vi "RefreshSystemConfigurationUI.vi"(8 "error in (no error)":errorcluster, 11 "SystemSetup in":refnum<class "SystemSetup.lvclass">) -> (0 "error out":errorcluster, 3 "SystemSetup out":refnum<class "SystemSetup.lvclass">)   [LabVIEW 2019, in "SystemSetup.lvlib" / "SystemSetup.lvclass"]
uses:
  SystemSetup.lvclass
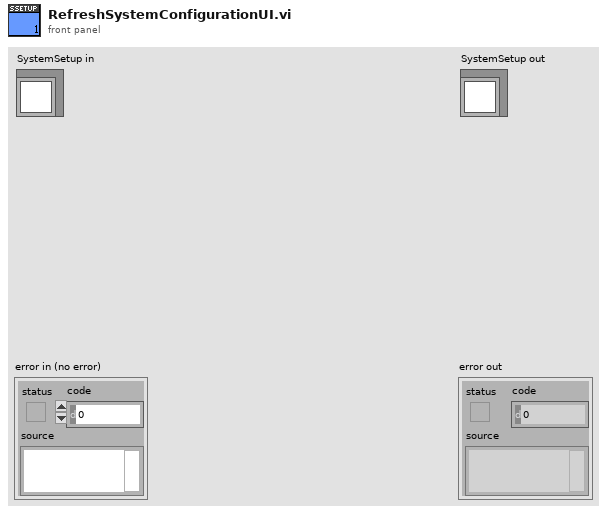
[diagram p1: front panel]
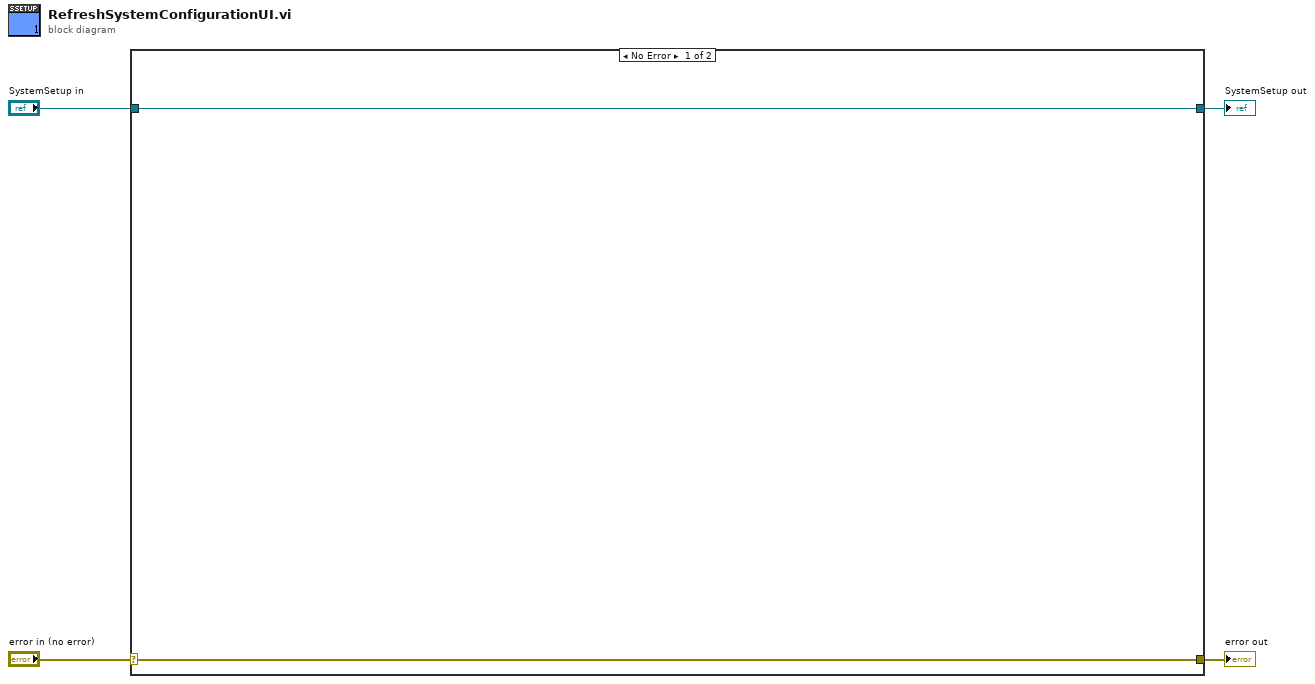
[diagram p0: block diagram]
diagram:
  n1 = case shown="No Error" "error in (no error)" {
    selector: "error in (no error)" -> [w5 w8]
    tunnel: [w5 w8] -> w3
    tunnel: [w6 w7] -> w1
    tunnel: "SystemSetup in" -> [w6 w7]
    frame No Error {
    }
    frame Error {
    }
  }
  "error out" <- w3
  "SystemSetup out" <- w1
